vi "Action Status to Text.vi"(1 "PSU Act Stat":T1) -> (0 "Status:":string)   [LabVIEW 2016, in "Instrument.Oxford1820.lvclass"]
uses:
  Instrument.Oxford1820.lvclass
  <instrlib>/Mercury iXX/Public/Libraries/Magnet/Controls/PSU Actions.ctl
  <instrlib>/Mercury iXX/Public/Libraries/Magnet.lvlib
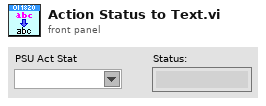
[diagram p1: front panel]
types:
  T1 = typedef "Mercury iXX.lvlib/Magnet.lvlib/PSU Actions.ctl" = string
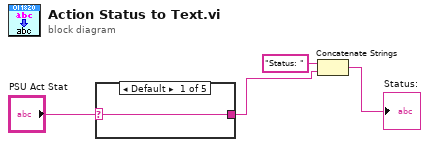
[diagram p0: block diagram]
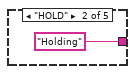
[diagram p2: hidden frame]
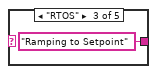
[diagram p3: hidden frame]
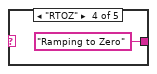
[diagram p4: hidden frame]
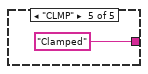
[diagram p5: hidden frame]
diagram:
  n1 = case shown="Default" "PSU Act Stat" {
    selector: "PSU Act Stat" -> [w5 _ _ _ _]
    tunnel: [w5 "Holding" "Ramping to Setpoint" "Ramping to Zero" "Clamped"] -> w2
    frame Default {
    }
    frame "HOLD" {
    }
    frame "RTOS" {
    }
    frame "RTOZ" {
    }
    frame "CLMP" {
    }
  }
  n2 = Concatenate Strings("Status: " ("string"), w2) -> (→"Status:":string)
